vi "Get Logger By Name.vi"(8 "error in (no error)":errorcluster, 10 "Name":string, 11 "Registry in":refnum<class "Registry.lvclass">) -> (0 "error out":errorcluster, 2 "Logger":refnum<class "Logger.lvclass">, 3 "Registry out":refnum<class "Registry.lvclass">)   [LabVIEW 2025, in "LV Logging.lvlib" / "Registry.lvclass"]
uses:
  Registry.lvclass
  Logger/Logger.lvclass
  Registry.lvclass/Registry.ctl
  <vilib>/ErrorRing/Error Ring.xnode
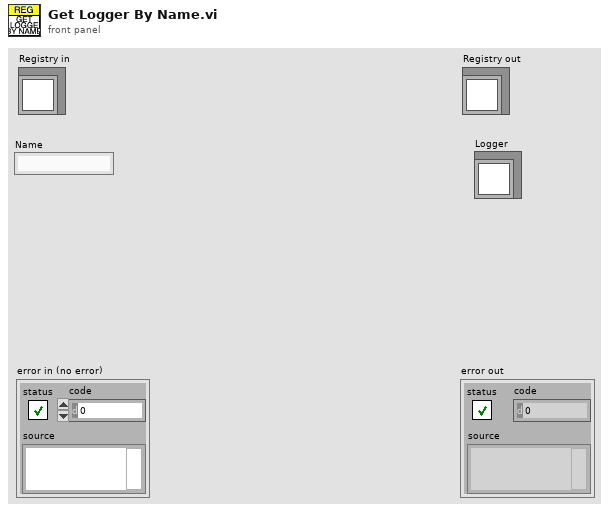
[diagram p1: front panel]
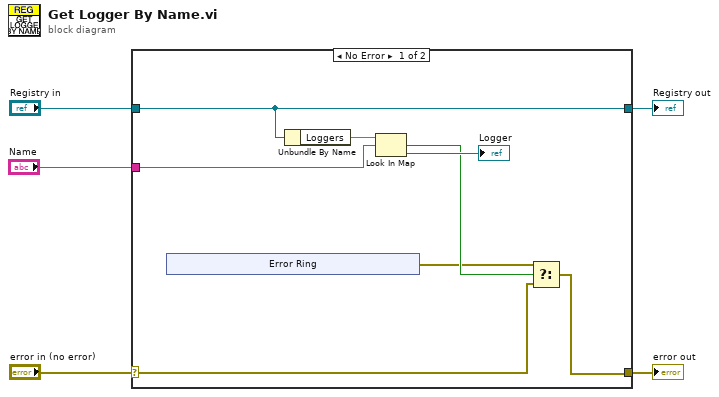
[diagram p0: block diagram]
diagram:
  n1 = case shown="No Error" "error in (no error)" {
    selector: "error in (no error)" -> [w7 w16]
    tunnel: [w8 w16] -> w4
    tunnel: [w13 w15] -> w2
    tunnel: "Registry in" -> [w13 w15]
    tunnel: "Name" -> [w11 _]
    frame No Error {
      n2 = xnode "Error Ring"() -> ("error out"=w6:errorcluster)
      n3 = Unbundle By Name(w13) -> ("Loggers"=w12:map{string, refnum<class "Logger.lvclass">})
      n4 = Look In Map(map=w12, key=w11) -> (key not found?=w9:bool, value=→"Logger":refnum<class "Logger.lvclass">)  [unwired: 1 in]
      n5 = Select(t=w6, s=w9, f=w7) -> (s? t:f=w8:errorcluster)
    }
    frame Error {
    }
  }
  "error out" <- w4
  "Registry out" <- w2
